vi "create object id.vi"(10 "instance id (0)":i32, 11 "class name":string) -> (3 "String":string)   [LabVIEW 2019, in "HLA Custom Device Shared.lvlib"]
uses:
  HLA Custom Device Shared.lvlib
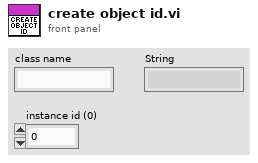
[diagram p1: front panel]
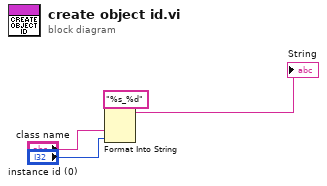
[diagram p0: block diagram]
diagram:
  n1 = Format Into String(format string="%s_%d", "class name", "instance id (0)") -> (resulting string=→"String":string)  [unwired: 2 in, 1 out]
